vi "Get cif_management_common_PluginStatusData.vi"(8 "error in (no error)":errorcluster, 11 "gRPCid":T1) -> (0 "error out":errorcluster, 2 "package_templatemessage":T2, 3 "gRPCid out":T1)   [LabVIEW 2021, in "CIF_PluginLoader_server.lvlib"]
uses:
  CIF_PluginLoader_server.lvlib
  cif_management_common_PluginStatusData.ctl
  cif_management_common_PluginStatusData_PluginState.ctl
  cif_management_common_TimingStatistics.ctl
  cif_common_TimingStats.ctl
  cif_management_common_FifoStatistics.ctl
  cif_management_common_Error.ctl
  cif_management_common_MonitorDoubles.ctl
  cif_management_common_MonitorU64.ctl
  cif_management_common_MonitorI64.ctl
  <vilib>/gRPC/LabVIEW gRPC Library/Shared/grpcId.ctl
  cif_management_common_PluginStatusData_Flat.ctl
  cif_management_common_TimingStatistics_Flat.ctl
  cif_common_TimingStats_Flat.ctl
  cif_management_common_FifoStatistics_Flat.ctl
  cif_management_common_Error_Flat.ctl
  cif_management_common_MonitorDoubles_Flat.ctl
  cif_management_common_MonitorU64_Flat.ctl
  cif_management_common_MonitorI64_Flat.ctl
  2ed25e12-861d-4677-8ead-ace2906b2041.vi
  <vilib>/gRPC/LabVIEW gRPC Library/Shared/TranslateGrpcError.vi
  FlatToRichcif_management_common_TimingStatistics.vi
  FlatToRichcif_management_common_FifoStatistics.vi
  FlatToRichcif_management_common_Error.vi
  FlatToRichcif_management_common_MonitorDoubles.vi
  FlatToRichcif_management_common_MonitorU64.vi
  FlatToRichcif_management_common_MonitorI64.vi
  FlatToRichcif_common_TimingStats.vi
  <vilib>/gRPC/LabVIEW gRPC Library/Server API/Server/Get Server DLL Path.vi
  <vilib>/Utility/error.llb/Error Cluster From Error Code.vi
  <vilib>/gRPC/LabVIEW gRPC Library/grpc-lvsupport-release.lvlib
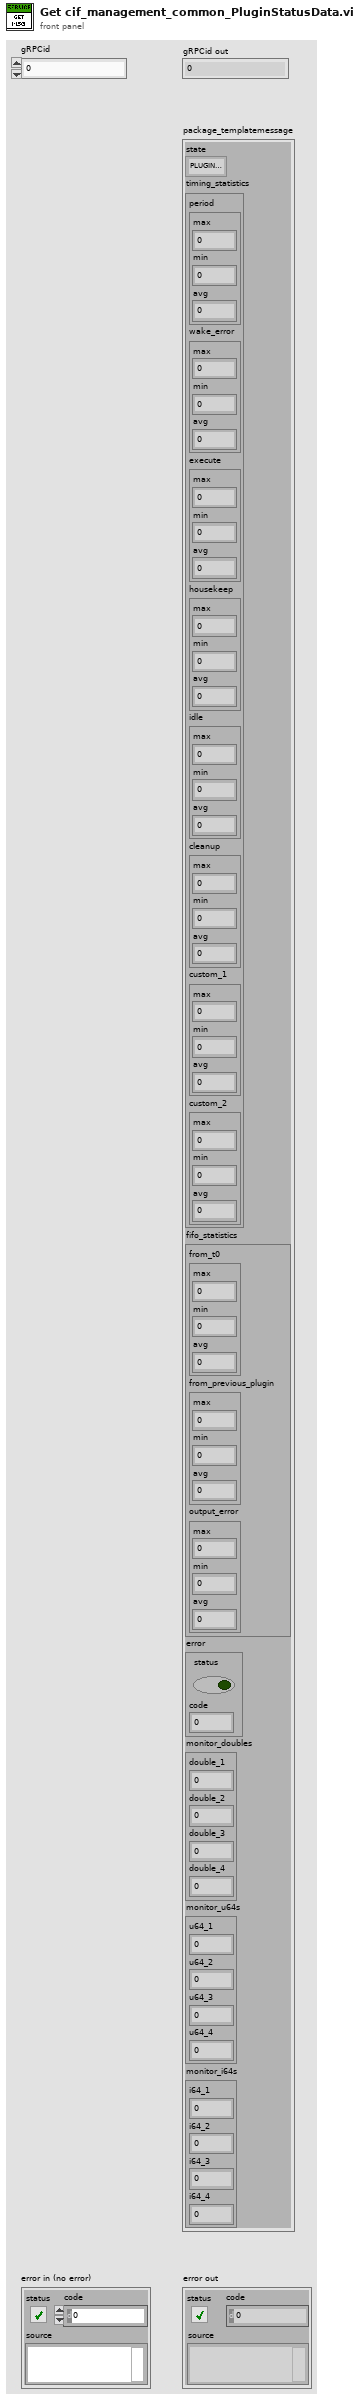
[diagram p1: front panel]
types:
  T1 = typedef "grpc-lvsupport-release.lvlib/grpcId.ctl" = u64
  T2 = typedef "CIF_PluginLoader_server.lvlib/cif_management_common_PluginStatusData.ctl" = cluster{"state":T3, "timing_statistics":T4, "fifo_statistics":T6, "error":T7, "monitor_doubles":T8, "monitor_u64s":T9, "monitor_i64s":T10}
  T3 = typedef "CIF_PluginLoader_server.lvlib/cif_management_common_PluginStatusData_PluginState.ctl" = enum32{"PLUGINSTATE_UNKNOWN", "PLUGINSTATE_CREATING", "PLUGINSTATE_LISTENING", "PLUGINSTATE_RUNNING", "PLUGINSTATE_CLEANINGUP", "PLUGINSTATE_DESTROYING", "PLUGINSTATE_PREPARED", "PLUGINSTATE_FTE_RUN"}
  T4 = typedef "CIF_PluginLoader_server.lvlib/cif_management_common_TimingStatistics.ctl" = cluster{"period":T5, "wake_error":T5, "execute":T5, "housekeep":T5, "idle":T5, "cleanup":T5, "custom_1":T5, "custom_2":T5}
  T5 = typedef "CIF_PluginLoader_server.lvlib/cif_common_TimingStats.ctl" = cluster{"max":i64, "min":i64, "avg":dbl}
  T6 = typedef "CIF_PluginLoader_server.lvlib/cif_management_common_FifoStatistics.ctl" = cluster{"from_t0":T5, "from_previous_plugin":T5, "output_error":T5}
  T7 = typedef "CIF_PluginLoader_server.lvlib/cif_management_common_Error.ctl" = cluster{"status":bool, "code":i32}
  T8 = typedef "CIF_PluginLoader_server.lvlib/cif_management_common_MonitorDoubles.ctl" = cluster{"double_1":dbl, "double_2":dbl, "double_3":dbl, "double_4":dbl}
  T9 = typedef "CIF_PluginLoader_server.lvlib/cif_management_common_MonitorU64.ctl" = cluster{"u64_1":u64, "u64_2":u64, "u64_3":u64, "u64_4":u64}
  T10 = typedef "CIF_PluginLoader_server.lvlib/cif_management_common_MonitorI64.ctl" = cluster{"i64_1":i64, "i64_2":i64, "i64_3":i64, "i64_4":i64}
  T11 = typedef "CIF_PluginLoader_server.lvlib/cif_management_common_PluginStatusData_Flat.ctl" = cluster{"state":T3, "timing_statistics":T12, "fifo_statistics":T14, "error":T15, "monitor_doubles":T16, "monitor_u64s":T17, "monitor_i64s":T18}
  T12 = typedef "CIF_PluginLoader_server.lvlib/cif_management_common_TimingStatistics_Flat.ctl" = cluster{"period":T13, "wake_error":T13, "execute":T13, "housekeep":T13, "idle":T13, "cleanup":T13, "custom_1":T13, "custom_2":T13}
  T13 = typedef "CIF_PluginLoader_server.lvlib/cif_common_TimingStats_Flat.ctl" = cluster{"max":i64, "min":i64, "avg":dbl}
  T14 = typedef "CIF_PluginLoader_server.lvlib/cif_management_common_FifoStatistics_Flat.ctl" = cluster{"from_t0":T13, "from_previous_plugin":T13, "output_error":T13}
  T15 = typedef "CIF_PluginLoader_server.lvlib/cif_management_common_Error_Flat.ctl" = cluster{"status":bool, "code":i32}
  T16 = typedef "CIF_PluginLoader_server.lvlib/cif_management_common_MonitorDoubles_Flat.ctl" = cluster{"double_1":dbl, "double_2":dbl, "double_3":dbl, "double_4":dbl}
  T17 = typedef "CIF_PluginLoader_server.lvlib/cif_management_common_MonitorU64_Flat.ctl" = cluster{"u64_1":u64, "u64_2":u64, "u64_3":u64, "u64_4":u64}
  T18 = typedef "CIF_PluginLoader_server.lvlib/cif_management_common_MonitorI64_Flat.ctl" = cluster{"i64_1":i64, "i64_2":i64, "i64_3":i64, "i64_4":i64}
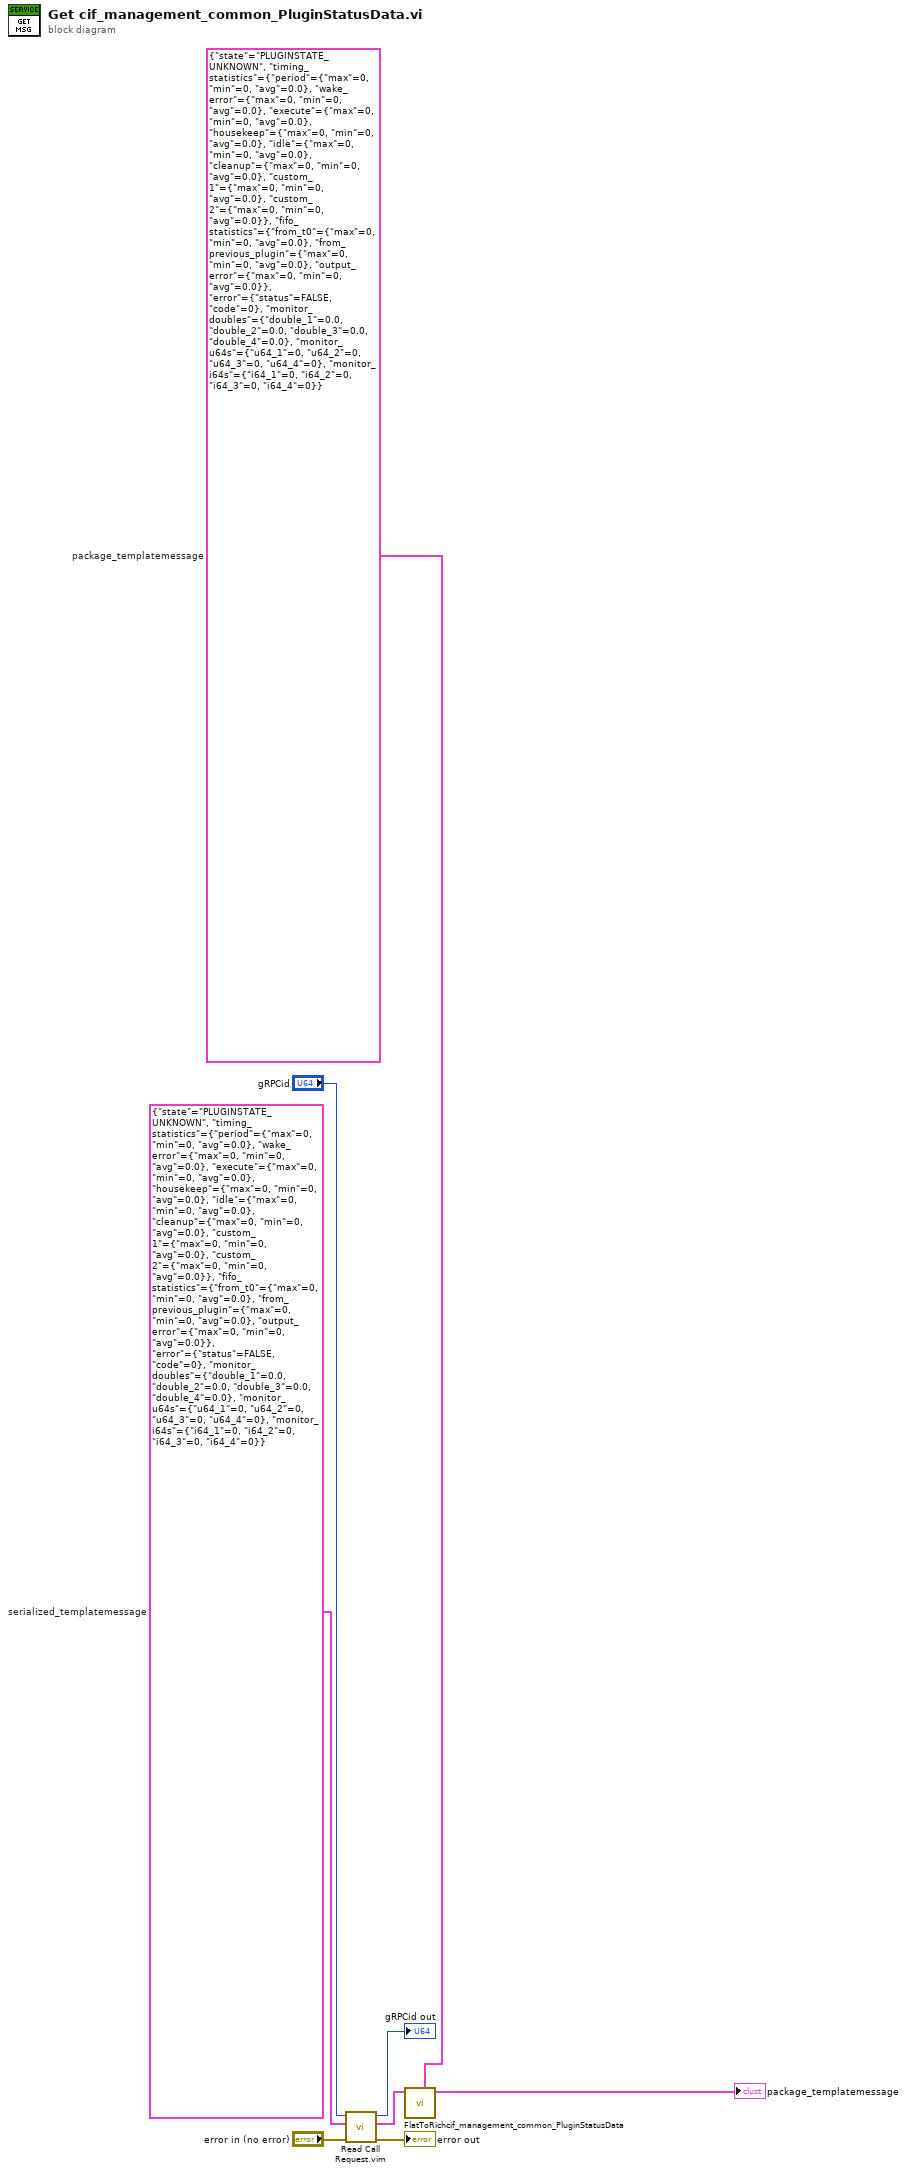
[diagram p0: block diagram]
diagram:
  w6 = T11 {"state"=enum."PLUGINSTATE_UNKNOWN", "timing_statistics"={"period"={"max"=0, "min"=0, "avg"=0.0}, "wake_error"={"max"=0, "min"=0, "avg"=0.0}, "execute"={"max"=0, "min"=0, "avg"=0.0}, "housekeep"={"max"=0, "min"=0, "avg"=0.0}, "idle"={"max"=0, "min"=0, "avg"=0.0}, "cleanup"={"max"=0, "min"=0, "avg"=0.0}, "custom_1"={"max"=0, "min"=0, "avg"=0.0}, "custom_2"={"max"=0, "min"=0, "avg"=0.0}}, "fifo_statistics"={"from_t0"={"max"=0, "min"=0, "avg"=0.0}, "from_previous_plugin"={"max"=0, "min"=0, "avg"=0.0}, "output_error"={"max"=0, "min"=0, "avg"=0.0}}, "error"={"status"=FALSE, "code"=0}, "monitor_doubles"={"double_1"=0.0, "double_2"=0.0, "double_3"=0.0, "double_4"=0.0}, "monitor_u64s"={"u64_1"=0, "u64_2"=0, "u64_3"=0, "u64_4"=0}, "monitor_i64s"={"i64_1"=0, "i64_2"=0, "i64_3"=0, "i64_4"=0}}  # serialized_templatemessage
  w5 = T2 {"state"=enum."PLUGINSTATE_UNKNOWN", "timing_statistics"={"period"={"max"=0, "min"=0, "avg"=0.0}, "wake_error"={"max"=0, "min"=0, "avg"=0.0}, "execute"={"max"=0, "min"=0, "avg"=0.0}, "housekeep"={"max"=0, "min"=0, "avg"=0.0}, "idle"={"max"=0, "min"=0, "avg"=0.0}, "cleanup"={"max"=0, "min"=0, "avg"=0.0}, "custom_1"={"max"=0, "min"=0, "avg"=0.0}, "custom_2"={"max"=0, "min"=0, "avg"=0.0}}, "fifo_statistics"={"from_t0"={"max"=0, "min"=0, "avg"=0.0}, "from_previous_plugin"={"max"=0, "min"=0, "avg"=0.0}, "output_error"={"max"=0, "min"=0, "avg"=0.0}}, "error"={"status"=FALSE, "code"=0}, "monitor_doubles"={"double_1"=0.0, "double_2"=0.0, "double_3"=0.0, "double_4"=0.0}, "monitor_u64s"={"u64_1"=0, "u64_2"=0, "u64_3"=0, "u64_4"=0}, "monitor_i64s"={"i64_1"=0, "i64_2"=0, "i64_3"=0, "i64_4"=0}}  # package_templatemessage
  n1 = call "Read Call Request.vim"("error in"="error in (no error)", "Request Type"=w6, "gRPCid in"="gRPCid") -> ("error out"=→"error out":errorcluster, "Request Data"=w4:T11, "gRPCid out"=→"gRPCid out":T1)  [unwired: 6 in]
  n2 = call "FlatToRichcif_management_common_PluginStatusData.vi"("OutputClusterType"=w5, "InputCluster"=w4) -> ("OutputCluster"=→"package_templatemessage":T2)  [unwired: 9 in]
